vi "TDMS_waform.vi"(9 "Timestamp":timestamp[](array[timestamp]), 10 "Current":dbl[](array[numeric]), 11 "Voltage":dbl[](array[numeric])) -> (3 "Array":waveform(dbl)[](array[waveform]))   [LabVIEW 2022 SP3]
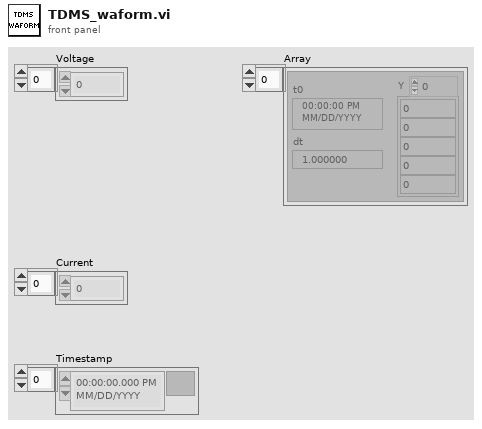
[diagram p1: front panel]
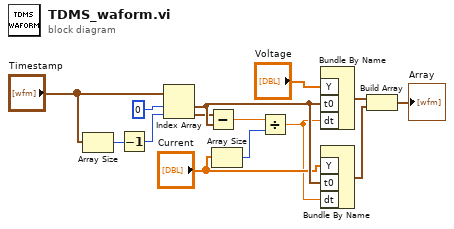
[diagram p0: block diagram]
diagram:
  n1 = Array Size(array="Timestamp") -> (size(s)=w6:i32)
  n2 = Decrement(x=w6) -> (x-1=w5:i32)
  n3 = Index Array(array="Timestamp", index #1=0 ("index"), index #2=w5) -> (element #1=w12:timestamp, element #2=w11:timestamp)
  n4 = Subtract(x=w11, y=w12) -> (x-y=w2:dbl)
  n5 = Array Size(array="Current") -> (size(s)=w3:i32)
  n6 = Divide(x=w2, y=w3) -> (x/y=w1:dbl)
  n7 = Bundle By Name("Y"="Voltage", "t0"=w12, "dt"=w1) -> (w14:waveform(dbl))  [unwired: 1 in]
  n8 = Bundle By Name("Y"="Current", "t0"=w12, "dt"=w1) -> (w13:waveform(dbl))  [unwired: 1 in]
  n9 = Build Array(w14, w13) -> (→"Array":waveform(dbl)[])
